vi "DebugBufferSpeedProfile.vi"(9 "positions":dbl[](array[numeric]), 10 "start":dbl, 11 "speed":dbl) -> (3 "speed history":T1(array[cluster]))   [LabVIEW 2017, in "CmsVirtualChannel.lvlib"]
uses:
  <vilib>/addons/InsightCM/Devices/Shared/Cms/CmsVirtualChannel/CmsVirtualChannel.lvlib
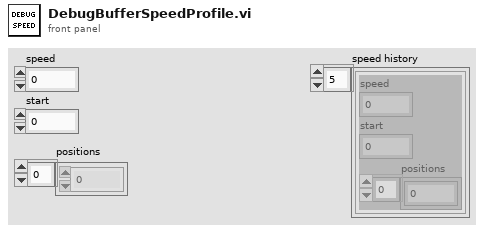
[diagram p1: front panel]
types:
  T1 = cluster{"speed":dbl, "start":dbl, "positions":dbl[]}[]
  T2 = cluster{"speed":dbl, "start":dbl, "positions":dbl[]}
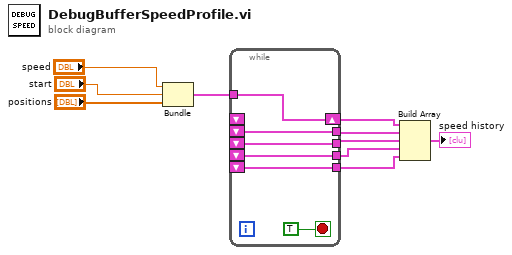
[diagram p0: block diagram]
diagram:
  n1 = Bundle("speed"="speed", "start"="start", "positions"="positions") -> (w6:T2)  [unwired: 1 in]
  n2 = while {
    shift-right: [w11] -> w5
    shift-left: _ -> [_]
    shift-left: _ -> [w15]
    shift-left: _ -> [w14]
    shift-left: _ -> [w13]
    shift-left: _ -> [w12]
    tunnel: [w15] -> w4
    tunnel: [w14] -> w3
    tunnel: [w13] -> w2
    tunnel: [w12] -> w1
    tunnel: w6 -> [w11]
    stop <- TRUE stop-if-true
  }
  n3 = Build Array(w5, w4, w3, w2, w1) -> (→"speed history":T1)
